vi "Set Tester Info.vi"(0 "TSM Context In":T1, 5 "Tester Type":string="RFPM", 7 "Resource Descriptors":string[](array[string]), 9 "Instrument Models":string[](array[string]), 11 "error in":errorcluster) -> (4 "TSM Context Out":T1, 15 "error out":errorcluster)   [LabVIEW 2023, in "RFCalAndFixtureCharact.Common.lvlib"]
uses:
  RFCalAndFixtureCharact.Common.lvlib
  <vilib>/NI_TestStand_SemiconductorModule/NI_TestStand_Semiconductor_Module.lvlibp/PinMap/General/SemiconductorModuleContext.ctl
  Global Data Id Prefix.vi
  <vilib>/NI_TestStand_SemiconductorModule/NI_TestStand_Semiconductor_Module.lvlibp
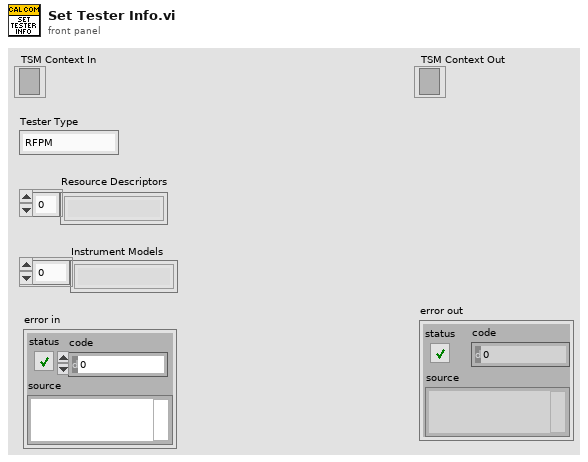
[diagram p1: front panel]
types:
  T1 = typedef "NI_TestStand_Semiconductor_Module.lvlibp/SemiconductorModuleContext.ctl" = refnum<k7>
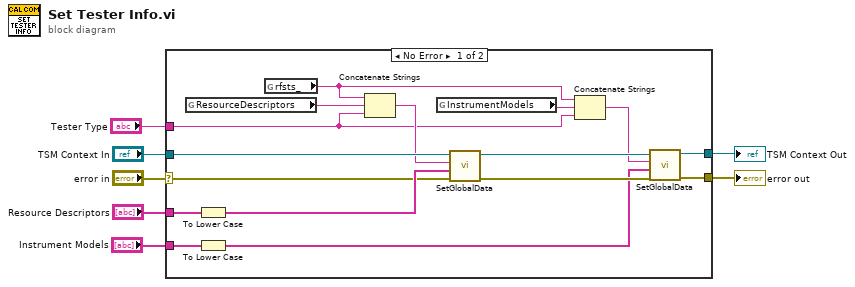
[diagram p0: block diagram]
diagram:
  n1 = case shown="No Error" "error in" {
    selector: "error in" -> [w13 w24]
    tunnel: "TSM Context In" -> [w23 w25]
    tunnel: "Resource Descriptors" -> [w22 _]
    tunnel: [w18 w24] -> w5
    tunnel: [w16 w25] -> w4
    tunnel: "Instrument Models" -> [w15 _]
    tunnel: "Tester Type" -> [w10 _]
    frame No Error {
      n2 = global read "Global Data Id Prefix.vi" "ResourceDescriptors"() -> (w9:string)
      n3 = To Lower Case(string=w22) -> (all lower case string=w20:string[])
      n4 = To Lower Case(string=w15) -> (all lower case string=w14:string[])
      n5 = global read "Global Data Id Prefix.vi" "rfsts_"() -> (w8:string)
      n6 = Concatenate Strings(w8, w9, w10) -> (w21:string)
      n7 = global read "Global Data Id Prefix.vi" "InstrumentModels"() -> (w12:string)
      n8 = call <vilib>:"SetGlobalData.vi"("error in (no error)"=w13, "Data"=w20, "Data Id"=w21, "Semiconductor Module Context"=w23) -> ("error out"=w19:errorcluster, "Semiconductor Module Context Out"=w17:T1)  [unwired: 5 in]
      n9 = Concatenate Strings(w8, w12, w10) -> (w11:string)
      n10 = call <vilib>:"SetGlobalData.vi"("error in (no error)"=w19, "Data"=w14, "Data Id"=w11, "Semiconductor Module Context"=w17) -> ("error out"=w18:errorcluster, "Semiconductor Module Context Out"=w16:T1)  [unwired: 5 in]
    }
    frame Error {
    }
  }
  "TSM Context Out" <- w4
  "error out" <- w5
